vi "Configuração.vi"() -> ()   [LabVIEW 2018]
uses:
  Global_Telescopio.vi
panel:
  in  "URL do finals2000A.all:":string
  in  "Case Constant\n(See Context Help) 4":bool
  in  "Case Constant\n(See Context Help)":bool
  out "error out":errorcluster
  in  "Geral":T1(tab)=enum."Pos. Cúpula"
  in  "wheather timeout":bool
  in  "Tempo sem dados":dbl=120.0 caption="segundos" min=0.0
  in  "PressãoMax":dbl=1200.0 caption="mbar"
  in  "UmidadeMax":dbl=100.0 caption="%"
  in  "TemperaturaMax":dbl=30.0 caption="ºC"
  in  "PressãoMin":dbl=500.0 caption="mbar"
  in  "UmidadeMin":dbl caption="%"
  in  "TemperaturaMin":dbl caption="ºC"
  in  "Salvar valores":bool
  in  "Pressão atmosférica":dbl=880.0 caption="mbar"
  in  "Umidade":dbl=88.0 caption="%"
  in  "Temperatura":dbl=15.0 caption="ºC"
  in  "Default Met":bool
  in  "Memorizar Default Met":bool
  in  "Caminho Estação Meteorológica":string="V 1.0.0 arquivo obsoleto. Usado apenas PUB ZeroMQ."
  in  "Desloc_Min_Cúpula":i32=2 min=2
  in  "OffsetCupula":dbl=135.0 format="%#_11g"
  in  "Salvar dados cupula":bool
  in  "OffsetZ":dbl=-0.28 format="%#_11g"
  in  "OffsetY":dbl format="%#_11g"
  in  "OffsetX":dbl format="%#_11g"
  in  "DistEixos":dbl=-0.62 format="%#_11g"
  in  "RaioCup":dbl=3.2 format="%#_11g"
  in  "LATrad":dbl=5.889885056 format="%#_11g"
  in  "Conf. Serial":bool
  in  "Aquisição":i32(ring) items=[" COM1", " COM2", " COM3", " COM4", " COM5", " COM6", " COM7", " COM8", " COM9", " COM10", " COM11", " COM12", " COM13", " COM14", " COM15", " COM16", " COM17", " COM18", " COM19", " COM20"]
  in  "Guider":i32(ring) items=[" COM1", " COM2", " COM3", " COM4", " COM5", " COM6", " COM7", " COM8", " COM9", " COM10", " COM11", " COM12", " COM13", " COM14", " COM15", " COM16", " COM17", " COM18", " COM19", " COM20"]
  in  "Teclado":i32(ring) items=[" COM1", " COM2", " COM3", " COM4", " COM5", " COM6", " COM7", " COM8", " COM9", " COM10", " COM11", " COM12", " COM13", " COM14", " COM15", " COM16", " COM17", " COM18", " COM19", " COM20"]
  out "Calagem DEC":string
  out "Calagem AH":string
  in  "LoadCalagem":bool
  in  "Instrumento":u16(ring) items=["Coude A+", "Coude B+", "ECass+", "Eucalyptus+", "Cam 1+", "Cam 2*", "Cam4 + IV*", "Polarimetro*", "Fortrap*", "Cam1 RF*", "Coude C+", "MUSICOS*", "+Já testado", "* nao config", "cam 1 s/rf", "cam1srf/luca+focali", "Coude A/luca", "ECass/luca", "Cam1+rf+luca", "MUSICOS+Luca", "Camiv+Luca", "Cam2+Luca", "Cam1+rf+luca+Ixon", "Cam1+rf+luca+Ikon", "CoudeTeste"]
  in  "Conf. Instrumentos":bool
  in  "Tabela Instrumentos":string[][](table)=[["Coude", "281.52", " 11.53", "S", "S", "0.462", "23.1", "23.1"], ["Cassegrain", "281.52", " 11.53", "S", "S", "0.462", "23.1", "23.1"], ["Eucalyptus", "281.52", " 11.53", "S", "S", "0.462", "23.1", "23.1"], ["Cam 1", "281.52", " 11.53", "S", "S", "0.462", "23.1", "23.1"], ["Cam 2", "281.52", " 11.53", "S", "S", "0.462", "23.1", "23.1"], ["Cam IV", "281.52", " 11.53", "S", "S", "0.462", "23.1", "23.1"], ["Polarimetro", "281.52", " 11.53", "S", "S", "0.462", "23.1", "23.1"], ["Fortrap", "281.52", " 11.53", "S", "S", "0.462", "23.1", "23.1"]]
  in  "CorrecaoMin":dbl=0.1
  in  "tel_sts1":bool[](array[boolean])=[TRUE, TRUE, TRUE, TRUE, FALSE, FALSE, TRUE]
  in  "Senha LEAF":string
  in  "Enable ventilador":bool=TRUE
  in  "habilita supervisao":bool
  in  "Tempo delay":i32=1
  in  "Limite Oeste":dbl=5.0 min=-12.0 max=12.0 step=0.1
  in  "Limite Leste":dbl=-4.5 min=-12.0 max=12.0 step=0.1
  out "DownloadWait":bool
  out "DownloadOK":bool caption="OK"
  in  "Download_Finals2000A.all":bool
  in  "Tempo Atualização All Sky":i32=1 min=1
  in  "Tempo Atualização Cam 3":i32=1 min=1
  in  "Tempo Atualização Cam 2":i32=1 min=1
  in  "Tempo Atualização Cam 1":i32=1 min=1
  in  "Tempo Atualização Cam 0":i32=1 min=1
  out "Ângulo Zenital":dbl format="%#.1f"
  out "Azimute":dbl format="%#.1f"
  in  "Tabela Proteção":string[][](table)=[["0", "360", "70", "60", "65"]]
  in  "Raio Máximo":dbl=5.0 min=0.0 max=90.0 step=0.1
  in  "Z_Max":dbl
  in  "Z_Libera":dbl
  in  "Z_Segurança":dbl
  in  "Hour Angle":string="00 00 0,00" caption="Dest AH"
  in  "Dest Dec":string="00 00 00,00"
  in  "SALVA CONFIG":bool
  out "DestDEC":dbl
  in  "DestCUP":i32
  out "DestAH":dbl
  in  "Caminho camera":string
  in  "Hora vent inicial":i32=1 min=0 max=86399 step=1 format="%<%H:%M:%S>t"
  in  "Hora vent final":i32=1 min=0 max=86399 step=1 format="%<%H:%M:%S>t"
  in  "ENGENHARIA":bool
  # "Configuração do Sistema"
  # "Caminho completo da Estação Meteorológica\nEx: http://200.131.64.185/clima/download.txt"
  # "Especifica o tempo para sinalizar que o TCSPD não está\nrecebendo os dados da estação meteorológica."
  # "Usar valores default se ocorrer a sinalização descrita acima."
  # "Valores Médios"
  # "Limite Mínimo"
  # "Limite Máximo"
  # "Quando \"Default Met\" for selecionado, sempre serão usados os valores médios (default) de temperatura, umidade e pressão atmosférica no cálculo da refração atmostérica e não os valores lidos da estação meteorológica, mesmo que estes sejam válidos e corretos."
  # "Se alguma leitura da estação meteorológica estiver fora dos limites acima, aquele valor será automaticamente substituído pelo seu valor médio."
  # "CONSTANTES DA CÚPULA"
  # "1,60m"
  # "IAG"
  # "5,889885056"
  # "5,889885056"
  # "7,525"
  # "3,20"
  # "-0,62"
  # "1,570"
  # "0,000"
  # "0,000"
  # "0,000"
  # "0,000"
  # "0,300"
  # "-0,28"
  # "136,0"
  # "-135,0"
  # "4"
  # "2"
  # "Valores default para o IAG (03/03/2011)"
  # "Ao precionar as Teclas de Captura\né necessário selecionar  a Região \nde interesse da imagem!"
  # "Selecione a Captrua\na ser posicionada"
  # "Seriais\nAuto Guider"
  # "Ângulo\nRotator"
  # "Ângulo\nNorte"
  # "Img.\nEsp."
  # "No\nCass."
  # "Escala\nPlaca"
  # "Calagem\nAH (\")"
  # "Calagem\nDEC (\")"
  # "Posição\nFoco"
  # "Escolha do Instrumento"
  # "Instrumento"
  # "Calagem"
  # "Carrega a calagem do telescópio com a calagem inicial do instrumento"
  # "CorrecaoMin: Valor em arcsec utilizado como limite para mover os\neixos AH e DEC nos processos de guiagem automática (auto-guider)\ne de offset do sistema de aquisição. Não será executado nenhum \nmovimento desses processos com deslocamento inferior a CorrecaoMin."
  # "Parâmetros PARK"
  # "Radianos"
  # "-->"
  # "Faixa do Azimute\n   De:              Ate:"
  # "Ângulo Zenital\n  Máx:       Segur.:       Libera:"
  # "-->"
  # "Raio da Calagem Local"
  # "Graus"
  # "Tempo de delay de comunicação"
  # "Arquivo finals2000A.all para precessão"
  # "Habilita Supervisão do Controlador"
  # "Horas"
  # "Horas"
  # "C:\\TCS\\ARQUIVOS\\finals2000A.all,  2,2Mb"
  # "Ventilador"
  # "Endereço da câmera"
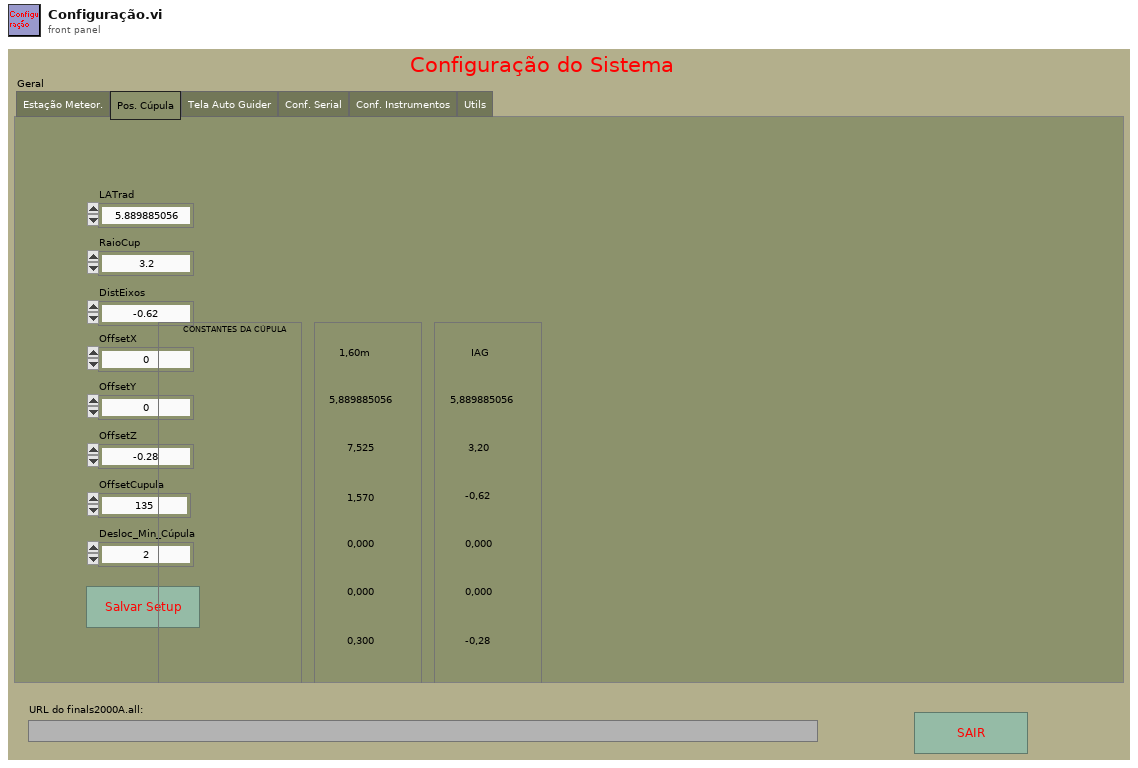
[diagram p1: front panel]
types:
  T1 = enum32{"Estação Meteor.", "Pos. Cúpula", "Tela Auto Guider", "Conf. Serial", "Conf. Instrumentos", "Utils"}
  T2 = cluster{"temperatura":dbl, "umidade":dbl, "pressao":dbl, "temperaturaMin":dbl, "umidadeMin":dbl, "pressaoMin":dbl, "temperaturaMax":dbl, "umidadeMax":dbl, "pressaoMax":dbl, "tempoSemDados":dbl}
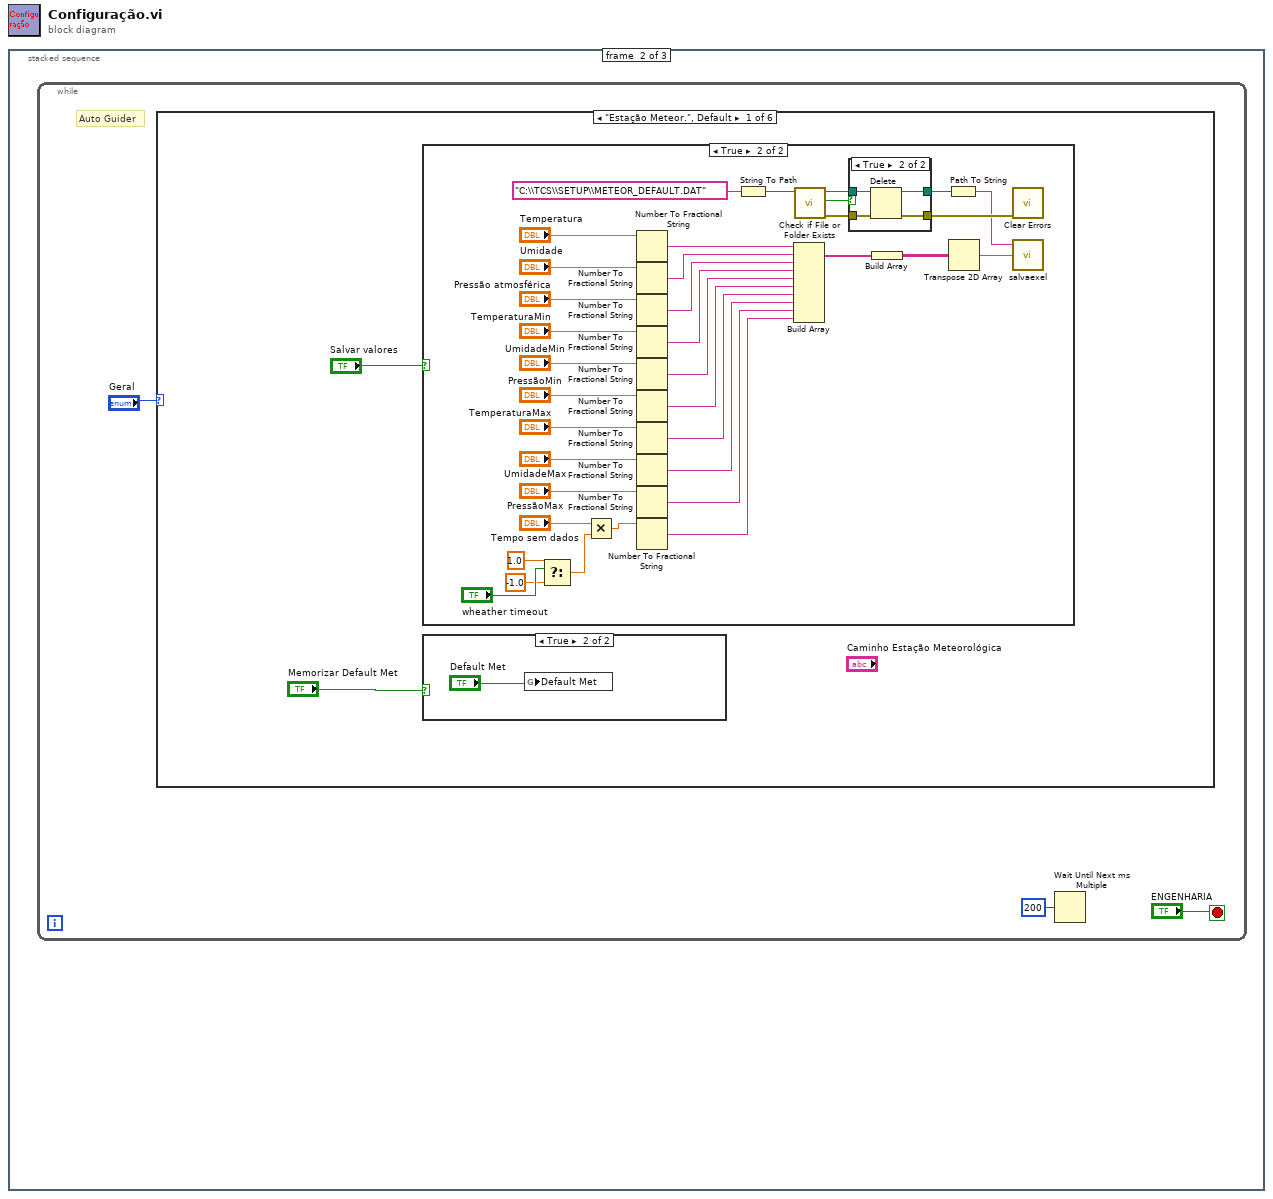
[diagram p0: block diagram]
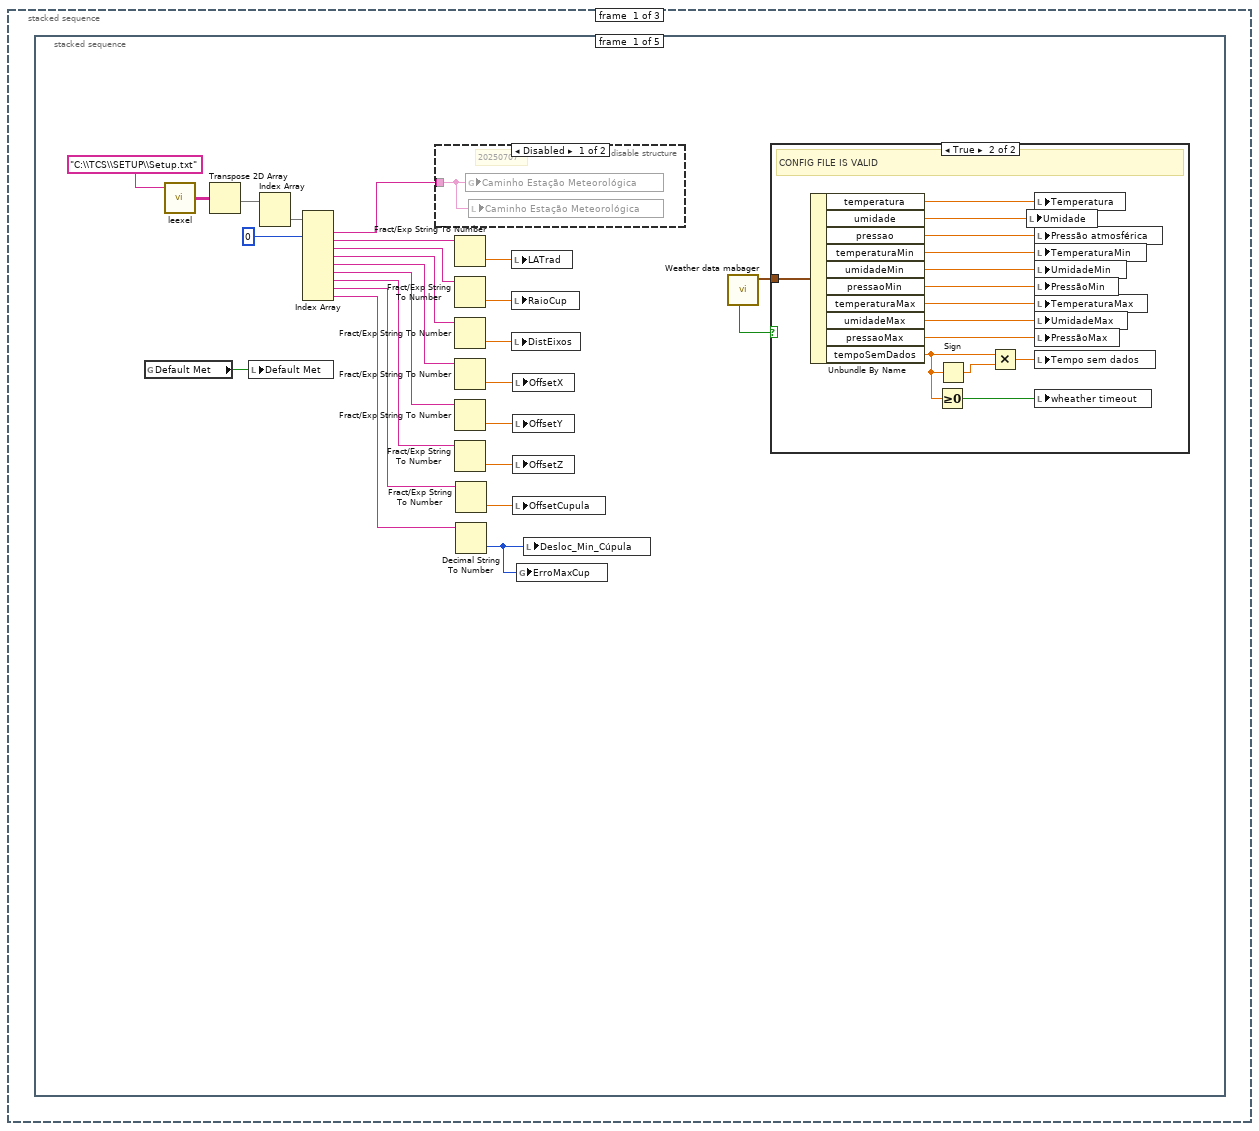
[diagram p2: hidden frame]
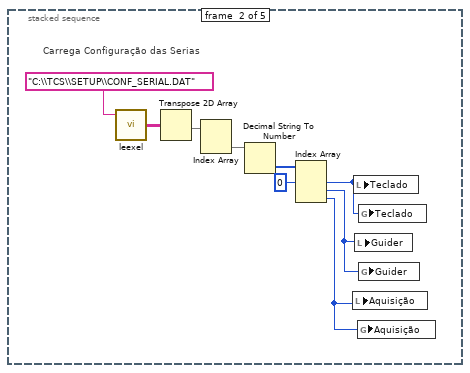
[diagram p5: hidden frame]
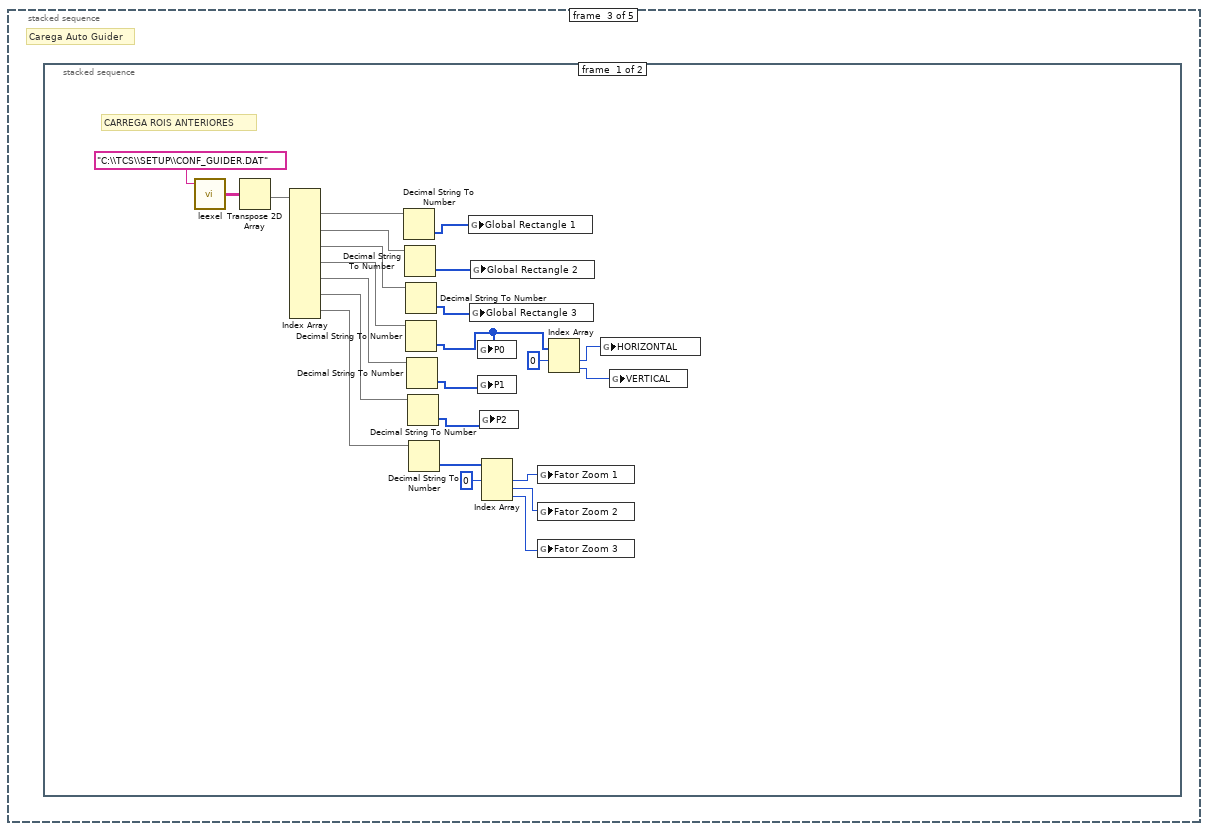
[diagram p6: hidden frame]
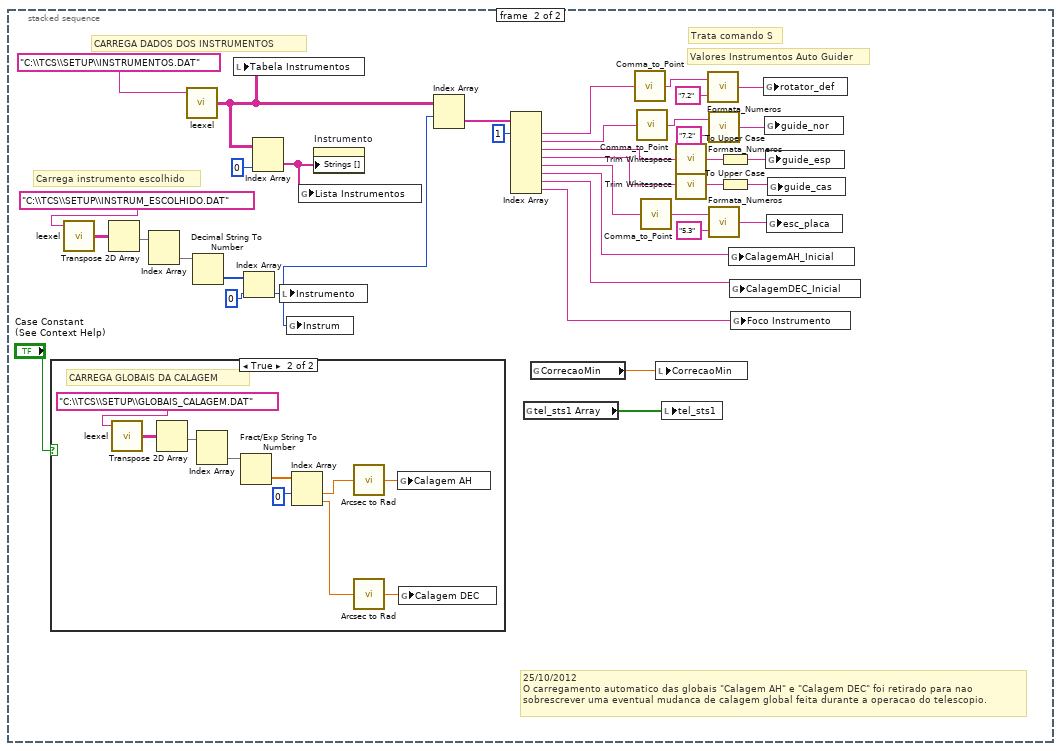
[diagram p7: hidden frame]
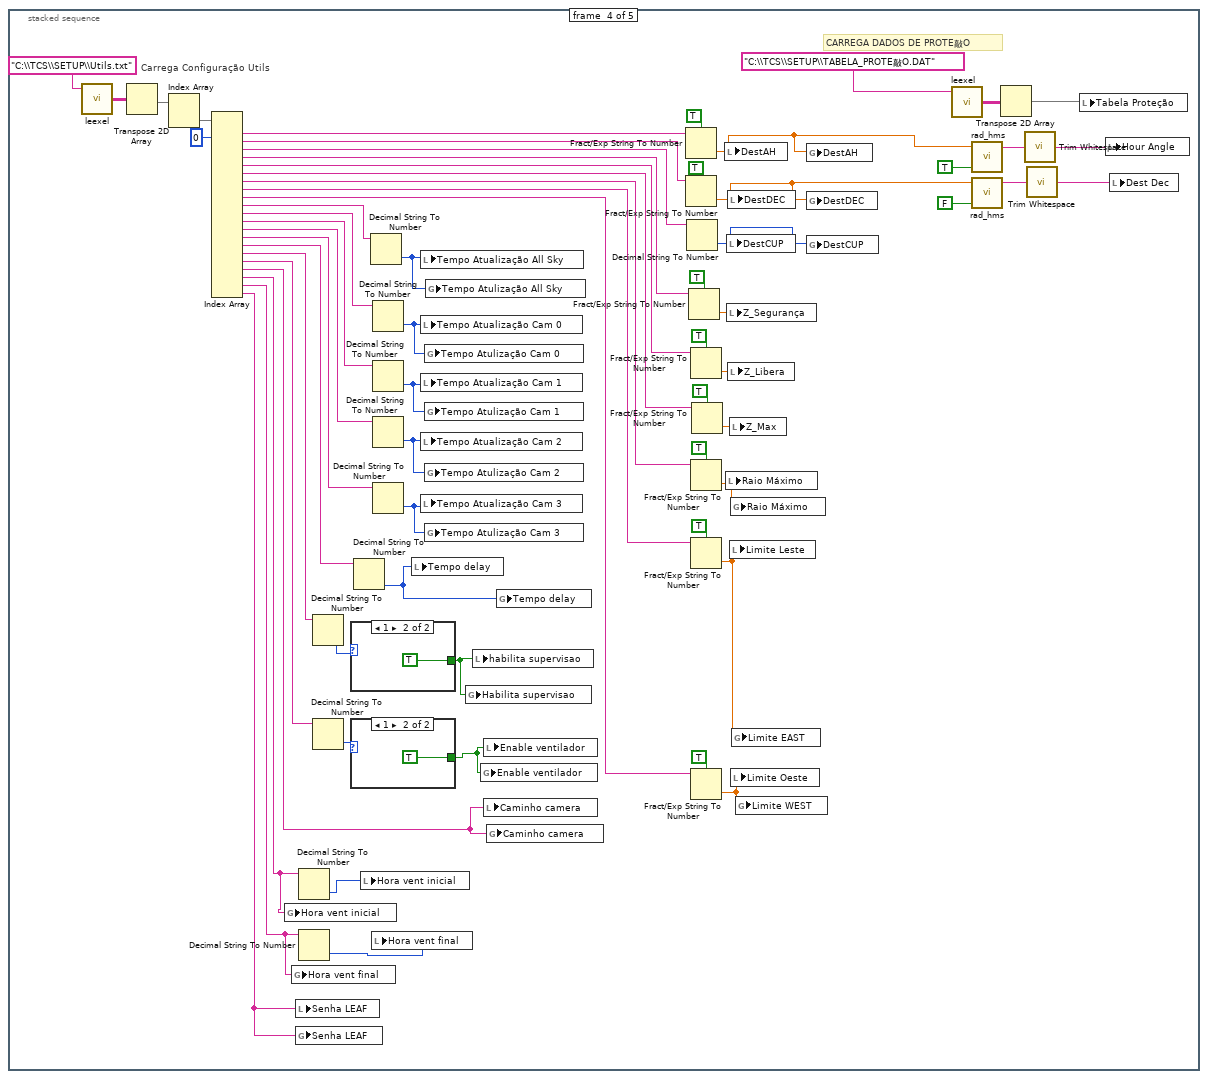
[diagram p9: hidden frame]
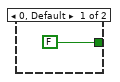
[diagram p10: hidden frame]
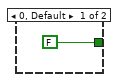
[diagram p11: hidden frame]
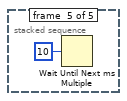
[diagram p12: hidden frame]
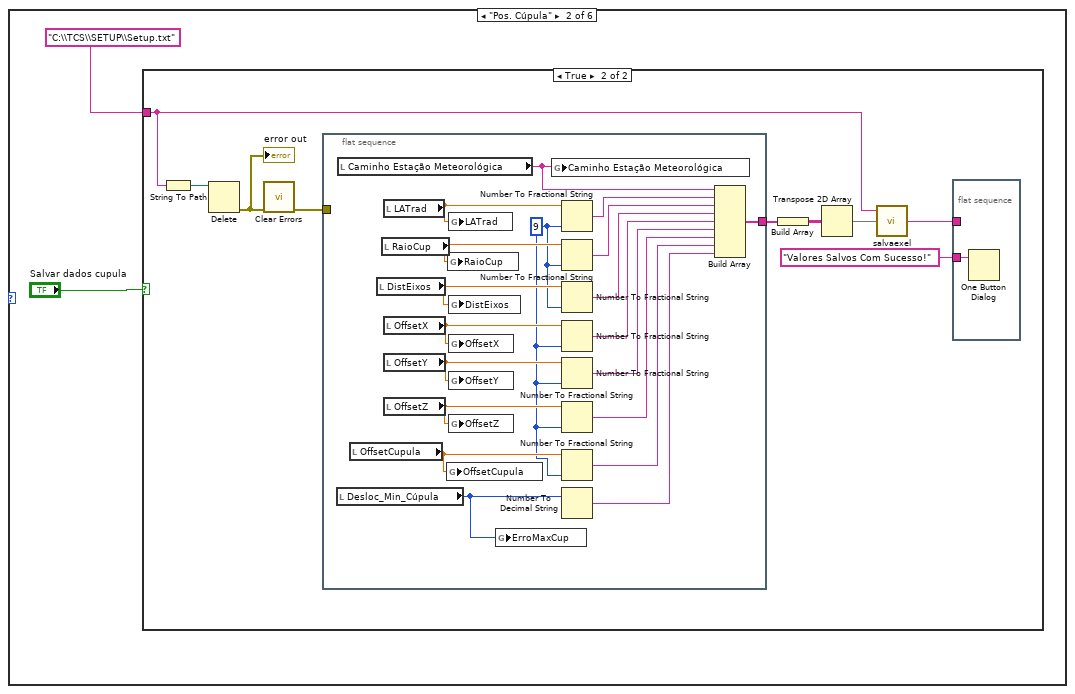
[diagram p16: hidden frame]
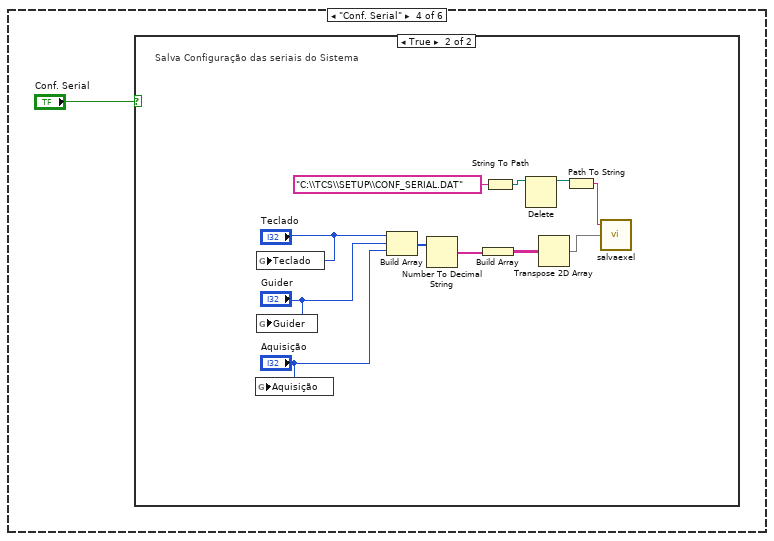
[diagram p19: hidden frame]
diagram:
  n1 = stacked-sequence {
    frame #0 {
      n2 = stacked-sequence {
        frame #0 {
          n3 = global read "Global_Telescopio.vi" "Default Met"() -> (w3:bool)
          n4 = call "leexel.vi"("path"="C:\\TCS\\SETUP\\Setup.txt") -> ("array 5"=w24:string[][])  [unwired: 4 in]
          n5 = Transpose 2D Array(2D array=w24) -> (transposed array=w23:string[][])
          n6 = local write "Default Met"(w3) -> ()
          n7 = Index Array(array=w23) -> (element=w22:string[])  [unwired: 2 in]
          n8 = Index Array(array=w22, index #1=0 ("index")) -> (element #1=w20:string, element #2=w18:string, element #3=w12:string, element #4=w11:string, element #5=w10:string, element #6=w9:string, element #7=w8:string, element #8=w6:string, element #9=w5:string)  [unwired: 8 in]
          n9 = disable-structure shown="Disabled" {
            disable-tunnel: w20 -> [w40 _]
            frame Disabled {
              # "20250707"
              n10 = global write "Global_Telescopio.vi" "Caminho Estação Meteorológica"(w40) -> ()
              n11 = local write "Caminho Estação Meteorológica"(w40) -> ()
            }
            frame Enabled {
            }
          }
          n12 = Fract/Exp String To Number(string=w18) -> (number=w19:dbl)  [unwired: 3 in, 1 out]
          n13 = Fract/Exp String To Number(string=w12) -> (number=w17:dbl)  [unwired: 3 in, 1 out]
          n14 = Fract/Exp String To Number(string=w11) -> (number=w16:dbl)  [unwired: 3 in, 1 out]
          n15 = Fract/Exp String To Number(string=w10) -> (number=w15:dbl)  [unwired: 3 in, 1 out]
          n16 = Fract/Exp String To Number(string=w9) -> (number=w14:dbl)  [unwired: 3 in, 1 out]
          n17 = Fract/Exp String To Number(string=w8) -> (number=w13:dbl)  [unwired: 3 in, 1 out]
          n18 = Fract/Exp String To Number(string=w6) -> (number=w7:dbl)  [unwired: 3 in, 1 out]
          n19 = Decimal String To Number(string=w5) -> (number=w4:i32)  [unwired: 2 in, 1 out]
          n20 = local write "LATrad"(w19) -> ()
          n21 = local write "RaioCup"(w17) -> ()
          n22 = local write "DistEixos"(w16) -> ()
          n23 = local write "OffsetX"(w15) -> ()
          n24 = local write "OffsetY"(w14) -> ()
          n25 = local write "OffsetZ"(w13) -> ()
          n26 = local write "OffsetCupula"(w7) -> ()
          n27 = global write "Global_Telescopio.vi" "ErroMaxCup"(w4) -> ()
          n28 = local write "Desloc_Min_Cúpula"(w4) -> ()
          n29 = call "Weather data mabager.vi"() -> ("weatherDefault"=w2:T2, "valid file"=w1:bool)  [unwired: 4 in, 6 out]
          n30 = case shown="True" w1 {
            tunnel: w2 -> [_ w39]
            frame False {
              # "INVALID CONFIG FILE - DOES NOT CHANGE DEFAULT CONTROL VALUES"
            }
            frame True {
              # "CONFIG FILE IS VALID"
              n31 = Unbundle By Name(w39) -> ("temperatura"=w38:dbl, "umidade"=w37:dbl, "pressao"=w36:dbl, "temperaturaMin"=w35:dbl, "umidadeMin"=w34:dbl, "pressaoMin"=w33:dbl, "temperaturaMax"=w32:dbl, "umidadeMax"=w31:dbl, "pressaoMax"=w30:dbl, "tempoSemDados"=w28:dbl)
              n32 = Greater Or Equal To 0?(x=w28) -> (x >= 0?=w29:bool)
              n33 = Sign(1:w28) -> (0:w27:dbl)
              n34 = Multiply(x=w28, y=w27) -> (x*y=w26:dbl)
              n35 = local write "Umidade"(w37) -> ()
              n36 = local write "Temperatura"(w38) -> ()
              n37 = local write "Pressão atmosférica"(w36) -> ()
              n38 = local write "TemperaturaMin"(w35) -> ()
              n39 = local write "UmidadeMin"(w34) -> ()
              n40 = local write "PressãoMin"(w33) -> ()
              n41 = local write "TemperaturaMax"(w32) -> ()
              n42 = local write "UmidadeMax"(w31) -> ()
              n43 = local write "PressãoMax"(w30) -> ()
              n44 = local write "Tempo sem dados"(w26) -> ()
              n45 = local write "wheather timeout"(w29) -> ()
            }
          }
        }
        frame #1 {
          # "Carrega Configuração das Serias"
          n46 = call "leexel.vi"("path"="C:\\TCS\\SETUP\\CONF_SERIAL.DAT") -> ("array 5"=w48:string[][])  [unwired: 4 in]
          n47 = Transpose 2D Array(2D array=w48) -> (transposed array=w47:string[][])
          n48 = Index Array(array=w47) -> (element=w49:string[])  [unwired: 2 in]
          n49 = Decimal String To Number(string=w49) -> (number=w45:i32[])  [unwired: 2 in, 1 out]
          n50 = Index Array(array=w45, index #1=0 ("index")) -> (element #1=w43:i32, element #2=w42:i32, element #3=w41:i32)  [unwired: 2 in]
          n51 = local write "Aquisição"(w41) -> ()
          n52 = local write "Teclado"(w43) -> ()
          n53 = local write "Guider"(w42) -> ()
          n54 = global write "Global_Telescopio.vi" "Aquisição"(w41) -> ()
          n55 = global write "Global_Telescopio.vi" "Teclado"(w43) -> ()
          n56 = global write "Global_Telescopio.vi" "Guider"(w42) -> ()
        }
        frame #2 {
          # "Carega Auto Guider"
          n57 = stacked-sequence {
            frame #0 {
              # "CARREGA ROIS ANTERIORES"
              n58 = call "leexel.vi"("path"="C:\\TCS\\SETUP\\CONF_GUIDER.DAT") -> ("array 5"=w72:string[][])  [unwired: 4 in]
              n59 = Transpose 2D Array(2D array=w72) -> (transposed array=w71:string[][])
              n60 = Index Array(array=w71) -> (element #1=w70:string[], element #2=w69:string[], element #3=w68:string[], element #4=w67:string[], element #5=w66:string[], element #6=w65:string[], element #7=w53:string[])  [unwired: 14 in]
              n61 = Decimal String To Number(string=w70) -> (number=w56:i32[])  [unwired: 2 in, 1 out]
              n62 = Decimal String To Number(string=w69) -> (number=w57:i32[])  [unwired: 2 in, 1 out]
              n63 = Decimal String To Number(string=w68) -> (number=w58:i32[])  [unwired: 2 in, 1 out]
              n64 = Decimal String To Number(string=w67) -> (number=w61:i32[])  [unwired: 2 in, 1 out]
              n65 = Decimal String To Number(string=w66) -> (number=w60:i32[])  [unwired: 2 in, 1 out]
              n66 = Decimal String To Number(string=w65) -> (number=w59:i32[])  [unwired: 2 in, 1 out]
              n67 = Decimal String To Number(string=w53) -> (number=w52:i32[])  [unwired: 2 in, 1 out]
              n68 = global write "Global_Telescopio.vi" "Global Rectangle 1"(w56) -> ()
              n69 = global write "Global_Telescopio.vi" "Global Rectangle 3"(w58) -> ()
              n70 = global write "Global_Telescopio.vi" "Global Rectangle 2"(w57) -> ()
              n71 = global write "Global_Telescopio.vi" "P0"(w61) -> ()
              n72 = global write "Global_Telescopio.vi" "P1"(w60) -> ()
              n73 = global write "Global_Telescopio.vi" "P2"(w59) -> ()
              n74 = Index Array(array=w52, index #1=0 ("index")) -> (element #1=w54:i32, element #2=w51:i32, element #3=w50:i32)  [unwired: 2 in]
              n75 = global write "Global_Telescopio.vi" "Fator Zoom 1"(w54) -> ()
              n76 = global write "Global_Telescopio.vi" "Fator Zoom 2"(w51) -> ()
              n77 = global write "Global_Telescopio.vi" "Fator Zoom 3"(w50) -> ()
              n78 = Index Array(array=w61, index #1=0 ("index")) -> (element #1=w63:i32, element #2=w62:i32)  [unwired: 1 in]
              n79 = global write "Global_Telescopio.vi" "HORIZONTAL"(w63) -> ()
              n80 = global write "Global_Telescopio.vi" "VERTICAL"(w62) -> ()
            }
            frame #1 {
              # "25/10/2012\nO carregamento automatico das globais \"Calagem AH\" e \"Calagem DEC\" foi retirado para nao \nsobrescrever uma eventual mudanca de calagem global feita durante a operacao do telescopio."
              # "Trata comando S"
              # "Valores Instrumentos Auto Guider"
              # "Carrega instrumento escolhido"
              # "CARREGA DADOS DOS INSTRUMENTOS"
              n81 = case shown="True" "Case Constant\n(See Context Help)" {
                frame False {
                }
                frame True {
                  # "CARREGA GLOBAIS DA CALAGEM"
                  n82 = call "leexel.vi"("path"="C:\\TCS\\SETUP\\GLOBAIS_CALAGEM.DAT") -> ("array 5"=w117:string[][])  [unwired: 4 in]
                  n83 = Transpose 2D Array(2D array=w117) -> (transposed array=w118:string[][])
                  n84 = Index Array(array=w118) -> (element=w116:string[])  [unwired: 2 in]
                  n85 = Fract/Exp String To Number(string=w116) -> (number=w120:dbl[])  [unwired: 3 in, 1 out]
                  n86 = Index Array(array=w120, index #1=0 ("index")) -> (element #1=w114:dbl, element #2=w113:dbl)  [unwired: 1 in]
                  n87 = call "Arcsec to Rad.vi"("Arcsec"=w114) -> ("rad"=w112:dbl)
                  n88 = call "Arcsec to Rad.vi"("Arcsec"=w113) -> ("rad"=w111:dbl)
                  n89 = global write "Global_Telescopio.vi" "Calagem AH"(w112) -> ()
                  n90 = global write "Global_Telescopio.vi" "Calagem DEC"(w111) -> ()
                }
              }
              n91 = call "leexel.vi"("path"="C:\\TCS\\SETUP\\INSTRUM_ESCOLHIDO.DAT") -> ("array 5"=w106:string[][])  [unwired: 4 in]
              n92 = Transpose 2D Array(2D array=w106) -> (transposed array=w105:string[][])
              n93 = Index Array(array=w105) -> (element=w107:string[])  [unwired: 2 in]
              n94 = call "leexel.vi"("path"="C:\\TCS\\SETUP\\INSTRUMENTOS.DAT") -> ("array 5"=w102:string[][])  [unwired: 4 in]
              n95 = Decimal String To Number(string=w107) -> (number=w103:i32[])  [unwired: 2 in, 1 out]
              n96 = local write "Tabela Instrumentos"(w102) -> ()
              n97 = Index Array(array=w103, index=0) -> (element=w94:i32)
              n98 = Index Array(array=w102, index (col)=0 ("disabled index (col)")) -> (element=w95:string[])  [unwired: 1 in]
              n99 = local write "Instrumento"(w94) -> ()
              n100 = global write "Global_Telescopio.vi" "Instrum"(w94) -> ()
              n101 = global write "Global_Telescopio.vi" "Lista Instrumentos"(w95) -> ()
              n102 = property on="Instrumento" class="Ring (strict)"("Strings []"=w95) -> ()  [unwired: 2 in, 2 out]
              n103 = Index Array(array=w102, index (row)=w94) -> (element=w100:string[])  [unwired: 1 in]
              n104 = Index Array(array=w100, index #1=1 ("index")) -> (element #1=w90:string, element #2=w86:string, element #3=w83:string, element #4=w80:string, element #5=w76:string, element #6=w97:string, element #7=w96:string, element #8=w75:string)  [unwired: 7 in]
              n105 = global read "Global_Telescopio.vi" "tel_sts1 Array"() -> (w98:bool[])
              n106 = global read "Global_Telescopio.vi" "CorrecaoMin"() -> (w99:dbl)
              n107 = call "Comma_to_Point.vi"("Lat_A"=w90) -> ("Saída"=w91:string)
              n108 = call "Comma_to_Point.vi"("Lat_A"=w86) -> ("Saída"=w87:string)
              n109 = call "Comma_to_Point.vi"("Lat_A"=w76) -> ("Saída"=w77:string)
              n110 = local write "CorrecaoMin"(w99) -> ()
              n111 = local write "tel_sts1"(w98) -> ()
              n112 = call <vilib>:"Trim Whitespace.vi"("string"=w83) -> ("trimmed string"=w85:string)  [unwired: 1 in]
              n113 = call <vilib>:"Trim Whitespace.vi"("string"=w80) -> ("trimmed string"=w82:string)  [unwired: 1 in]
              n114 = call "Formata_Numeros.vi"("Formato ex-> 7.2"="7.2", "Valor num"=w91) -> ("resulting string"=w92:string)
              n115 = call "Formata_Numeros.vi"("Formato ex-> 7.2"="7.2", "Valor num"=w87) -> ("resulting string"=w88:string)
              n116 = call "Formata_Numeros.vi"("Formato ex-> 7.2"="5.3", "Valor num"=w77) -> ("resulting string"=w78:string)
              n117 = To Upper Case(1:w85) -> (0:w84:string)
              n118 = To Upper Case(1:w82) -> (0:w81:string)
              n119 = global write "Global_Telescopio.vi" "CalagemAH_Inicial"(w97) -> ()
              n120 = global write "Global_Telescopio.vi" "CalagemDEC_Inicial"(w96) -> ()
              n121 = global write "Global_Telescopio.vi" "Foco Instrumento"(w75) -> ()
              n122 = global write "Global_Telescopio.vi" "rotator_def"(w92) -> ()
              n123 = global write "Global_Telescopio.vi" "guide_nor"(w88) -> ()
              n124 = global write "Global_Telescopio.vi" "guide_esp"(w84) -> ()
              n125 = global write "Global_Telescopio.vi" "esc_placa"(w78) -> ()
              n126 = global write "Global_Telescopio.vi" "guide_cas"(w81) -> ()
            }
          }
        }
        frame #3 {
          # "CARREGA DADOS DE PROTE敲O"
          # "Carrega Configuração Utils"
          n127 = call "leexel.vi"("path"="C:\\TCS\\SETUP\\Utils.txt") -> ("array 5"=w183:string[][])  [unwired: 4 in]
          n128 = Transpose 2D Array(2D array=w183) -> (transposed array=w182:string[][])
          n129 = Index Array(array=w182) -> (element=w181:string[])  [unwired: 2 in]
          n130 = Index Array(array=w181, index #1=0 ("index")) -> (element #1=w179:string, element #2=w178:string, element #3=w177:string, element #4=w162:string, element #5=w161:string, element #6=w160:string, element #7=w154:string, element #8=w136:string, element #9=w135:string, element #10=w141:string, element #11=w142:string, element #12=w143:string, element #13=w144:string, element #14=w145:string, element #15=w134:string, element #16=w133:string, element #17=w126:string, element #18=w127:string, element #19=w122:string, element #20=w123:string, element #21=w121:string)  [unwired: 20 in]
          n131 = global write "Global_Telescopio.vi" "Hora vent inicial"(w122) -> ()
          n132 = global write "Global_Telescopio.vi" "Hora vent final"(w123) -> ()
          n133 = local write "Senha LEAF"(w121) -> ()
          n134 = global write "Global_Telescopio.vi" "Senha LEAF"(w121) -> ()
          n135 = Decimal String To Number(string=w122) -> (number=w125:i32)  [unwired: 2 in, 1 out]
          n136 = Decimal String To Number(string=w123) -> (number=w124:i32)  [unwired: 2 in, 1 out]
          n137 = Decimal String To Number(string=w133) -> (number=w132:i32)  [unwired: 2 in, 1 out]
          n138 = Decimal String To Number(string=w126) -> (number=w129:i32)  [unwired: 2 in, 1 out]
          n139 = case shown="1" w132 {
            tunnel: [FALSE TRUE] -> w131
            frame 0, Default {
            }
            frame 1 {
            }
          }
          n140 = case shown="1" w129 {
            tunnel: [FALSE TRUE] -> w128
            frame 0, Default {
            }
            frame 1 {
            }
          }
          n141 = Decimal String To Number(string=w134) -> (number=w130:i32)  [unwired: 2 in, 1 out]
          n142 = local write "Hora vent inicial"(w125) -> ()
          n143 = Decimal String To Number(string=w141) -> (number=w150:i32)  [unwired: 2 in, 1 out]
          n144 = local write "Hora vent final"(w124) -> ()
          n145 = Decimal String To Number(string=w142) -> (number=w149:i32)  [unwired: 2 in, 1 out]
          n146 = Decimal String To Number(string=w143) -> (number=w148:i32)  [unwired: 2 in, 1 out]
          n147 = Decimal String To Number(string=w144) -> (number=w147:i32)  [unwired: 2 in, 1 out]
          n148 = Decimal String To Number(string=w145) -> (number=w146:i32)  [unwired: 2 in, 1 out]
          n149 = local write "Tempo delay"(w130) -> ()
          n150 = local write "Tempo Atualização All Sky"(w150) -> ()
          n151 = local write "Tempo Atualização Cam 0"(w149) -> ()
          n152 = local write "Tempo Atualização Cam 1"(w148) -> ()
          n153 = local write "Tempo Atualização Cam 2"(w147) -> ()
          n154 = local write "Tempo Atualização Cam 3"(w146) -> ()
          n155 = global write "Global_Telescopio.vi" "Tempo Atulização Cam 0"(w149) -> ()
          n156 = global write "Global_Telescopio.vi" "Tempo Atulização Cam 1"(w148) -> ()
          n157 = global write "Global_Telescopio.vi" "Tempo Atulização Cam 2"(w147) -> ()
          n158 = global write "Global_Telescopio.vi" "Tempo Atulização Cam 3"(w146) -> ()
          n159 = global write "Global_Telescopio.vi" "Tempo Atulização All Sky"(w150) -> ()
          n160 = global write "Global_Telescopio.vi" "Habilita supervisao"(w131) -> ()
          n161 = local write "habilita supervisao"(w131) -> ()
          n162 = global write "Global_Telescopio.vi" "Enable ventilador"(w128) -> ()
          n163 = local write "Enable ventilador"(w128) -> ()
          n164 = local write "Caminho camera"(w127) -> ()
          n165 = global write "Global_Telescopio.vi" "Caminho camera"(w127) -> ()
          n166 = global write "Global_Telescopio.vi" "Tempo delay"(w130) -> ()
          n167 = Fract/Exp String To Number(use system decimal point (T)=TRUE, string=w179) -> (number=w173:dbl)  [unwired: 2 in, 1 out]
          n168 = Fract/Exp String To Number(use system decimal point (T)=TRUE, string=w178) -> (number=w172:dbl)  [unwired: 2 in, 1 out]
          n169 = Decimal String To Number(string=w177) -> (number=w176:i32)  [unwired: 2 in, 1 out]
          n170 = Fract/Exp String To Number(use system decimal point (T)=TRUE, string=w162) -> (number=w159:dbl)  [unwired: 2 in, 1 out]
          n171 = Fract/Exp String To Number(use system decimal point (T)=TRUE, string=w161) -> (number=w158:dbl)  [unwired: 2 in, 1 out]
          n172 = Fract/Exp String To Number(use system decimal point (T)=TRUE, string=w154) -> (number=w155:dbl)  [unwired: 2 in, 1 out]
          n173 = Fract/Exp String To Number(use system decimal point (T)=TRUE, string=w136) -> (number=w137:dbl)  [unwired: 2 in, 1 out]
          n174 = Fract/Exp String To Number(use system decimal point (T)=TRUE, string=w135) -> (number=w138:dbl)  [unwired: 2 in, 1 out]
          n175 = Fract/Exp String To Number(use system decimal point (T)=TRUE, string=w160) -> (number=w157:dbl)  [unwired: 2 in, 1 out]
          n176 = local write "DestAH"(w173) -> ()
          n177 = local write "Raio Máximo"(w155) -> ()
          n178 = local write "DestCUP"(w176) -> ()
          n179 = local write "Z_Segurança"(w159) -> ()
          n180 = local write "DestDEC"(w172) -> ()
          n181 = local write "Z_Libera"(w158) -> ()
          n182 = local write "Z_Max"(w157) -> ()
          n183 = local write "Limite Leste"(w137) -> ()
          n184 = global write "Global_Telescopio.vi" "Raio Máximo"(w155) -> ()
          n185 = local write "Limite Oeste"(w138) -> ()
          n186 = global write "Global_Telescopio.vi" "Limite EAST"(w137) -> ()
          n187 = global write "Global_Telescopio.vi" "Limite WEST"(w138) -> ()
          n188 = global write "Global_Telescopio.vi" "DestAH"(w173) -> ()
          n189 = global write "Global_Telescopio.vi" "DestDEC"(w172) -> ()
          n190 = global write "Global_Telescopio.vi" "DestCUP"(w176) -> ()
          n191 = call "leexel.vi"("path"="C:\\TCS\\SETUP\\TABELA_PROTE敲O.DAT") -> ("array 5"=w152:string[][])  [unwired: 4 in]
          n192 = call "rad_hms.vi"("TRUE=HORA\nFALSE=GRAU"=TRUE, "Radiano"=w173) -> ("Hora/Graus Texto Decimal"=w167:string)  [unwired: 3 in]
          n193 = call "rad_hms.vi"("TRUE=HORA\nFALSE=GRAU"=FALSE, "Radiano"=w172) -> ("Hora/Graus Texto Decimal"=w166:string)  [unwired: 3 in]
          n194 = Transpose 2D Array(2D array=w152) -> (transposed array=w151:string[][])
          n195 = call <vilib>:"Trim Whitespace.vi"("string"=w167) -> ("trimmed string"=w168:string)  [unwired: 1 in]
          n196 = call <vilib>:"Trim Whitespace.vi"("string"=w166) -> ("trimmed string"=w169:string)  [unwired: 1 in]
          n197 = local write "Tabela Proteção"(w151) -> ()
          n198 = local write "Hour Angle"(w168) -> ()
          n199 = local write "Dest Dec"(w169) -> ()
        }
        frame #4 {
          n200 = Wait Until Next ms Multiple(millisecond multiple=u32 10) -> ()  [unwired: 1 out]
        }
      }
    }
    frame #1 {
      n201 = while {
        stop <- "ENGENHARIA" stop-if-true
        # "Auto Guider"
        n202 = case shown="\"Estação Meteor.\", Default" "Geral" {
          frame "Estação Meteor.", Default {
            n203 = case shown="True" "Salvar valores" {
              frame False {
              }
              frame True {
                n204 = Select(t=1.0, s="wheather timeout", f=-1.0 ("t")) -> (s? t:f=w198:dbl)
                n205 = Multiply(x="Tempo sem dados", y=w198) -> (x*y=w200:dbl)
                n206 = Number To Fractional String(number="Temperatura") -> (F-format string=w229:string)  [unwired: 3 in]
                n207 = Number To Fractional String(number="Umidade") -> (F-format string=w228:string)  [unwired: 3 in]
                n208 = Number To Fractional String(number="Pressão atmosférica") -> (F-format string=w227:string)  [unwired: 3 in]
                n209 = Number To Fractional String(number="TemperaturaMin") -> (F-format string=w207:string)  [unwired: 3 in]
                n210 = Number To Fractional String(number="UmidadeMin") -> (F-format string=w206:string)  [unwired: 3 in]
                n211 = Number To Fractional String(number="PressãoMin") -> (F-format string=w205:string)  [unwired: 3 in]
                n212 = Number To Fractional String(number="TemperaturaMax") -> (F-format string=w204:string)  [unwired: 3 in]
                n213 = Number To Fractional String(number="UmidadeMax") -> (F-format string=w203:string)  [unwired: 3 in]
                n214 = Number To Fractional String(number="PressãoMax") -> (F-format string=w202:string)  [unwired: 3 in]
                n215 = Number To Fractional String(number=w200) -> (F-format string=w201:string)  [unwired: 3 in]
                n216 = String To Path(string="C:\\TCS\\SETUP\\METEOR_DEFAULT.DAT") -> (path=w220:path)
                n217 = Build Array(w229, w228, w227, w207, w206, w205, w204, w203, w202, w201) -> (w223:string[])
                n218 = call <vilib>:"Check if File or Folder Exists.vi"("path"=w220) -> ("error out"=w218:errorcluster, "file or folder exists?"=w217:bool, "dup path"=w219:path)  [unwired: 8 in]
                n219 = case shown="True" w217 {
                  tunnel: [w231 w236] -> w221
                  tunnel: w219 -> [w232 w235]
                  tunnel: w218 -> [w231 w234]
                  tunnel: [w232 w233] -> w216
                  frame False {
                  }
                  frame True {
                    n220 = Delete(path (use dialog)=w235, error in=w234) -> (deleted path=w233:path, error out=w236:errorcluster)  [unwired: 3 in, 1 out]
                  }
                }
                n221 = Build Array(w223) -> (w222:string[][])
                n222 = Path To String(path=w216) -> (string=w214:string)
                n223 = Transpose 2D Array(2D array=w222) -> (transposed array=w230:string[][])
                n224 = call <vilib>:"Clear Errors.vi"("error in (no error)"=w221) -> ()  [unwired: 5 in, 2 out]
                n225 = call "salvaexel.vi"("appended array"=w230, "file name p/ exell"=w214) -> ()  [unwired: 1 in, 1 out]
              }
            }
            n226 = case shown="True" "Memorizar Default Met" {
              frame False {
              }
              frame True {
                n227 = global write "Global_Telescopio.vi" "Default Met"("Default Met") -> ()
              }
            }
          }
          frame "Pos. Cúpula" {
            n228 = case shown="True" "Salvar dados cupula" {
              tunnel: "C:\\TCS\\SETUP\\Setup.txt" -> [_ w242]
              frame False {
              }
              frame True {
                n229 = String To Path(string=w242) -> (path=w248:path)
                n230 = Delete(path (use dialog)=w248) -> (error out=w247:errorcluster)  [unwired: 4 in, 2 out]
                "error out" <- w247
                n231 = call <vilib>:"Clear Errors.vi"("error in (no error)"=w247) -> ("error out"=w246:errorcluster)  [unwired: 5 in, 1 out]
                n232 = flat-sequence {
                  tunnel: w246 -> [_]
                  tunnel: [w251] -> w243
                  frame #0 {
                    w252 = i16 9 ("precision (6)")
                    n233 = local read "Desloc_Min_Cúpula"() -> (w260:i32)
                    n234 = local read "Caminho Estação Meteorológica"() -> (w250:string)
                    n235 = local read "OffsetCupula"() -> (w253:dbl)
                    n236 = local read "DistEixos"() -> (w257:dbl)
                    n237 = local read "RaioCup"() -> (w258:dbl)
                    n238 = local read "LATrad"() -> (w259:dbl)
                    n239 = local read "OffsetX"() -> (w256:dbl)
                    n240 = local read "OffsetY"() -> (w255:dbl)
                    n241 = local read "OffsetZ"() -> (w254:dbl)
                    n242 = global write "Global_Telescopio.vi" "OffsetCupula"(w253) -> ()
                    n243 = global write "Global_Telescopio.vi" "RaioCup"(w258) -> ()
                    n244 = global write "Global_Telescopio.vi" "LATrad"(w259) -> ()
                    n245 = global write "Global_Telescopio.vi" "DistEixos"(w257) -> ()
                    n246 = global write "Global_Telescopio.vi" "OffsetX"(w256) -> ()
                    n247 = global write "Global_Telescopio.vi" "OffsetY"(w255) -> ()
                    n248 = global write "Global_Telescopio.vi" "OffsetZ"(w254) -> ()
                    n249 = global write "Global_Telescopio.vi" "ErroMaxCup"(w260) -> ()
                    n250 = global write "Global_Telescopio.vi" "Caminho Estação Meteorológica"(w250) -> ()
                    n251 = Number To Fractional String(number=w259, precision (6)=w252) -> (F-format string=w268:string)  [unwired: 2 in]
                    n252 = Number To Fractional String(number=w258, precision (6)=w252) -> (F-format string=w267:string)  [unwired: 2 in]
                    n253 = Number To Fractional String(number=w257, precision (6)=w252) -> (F-format string=w266:string)  [unwired: 2 in]
                    n254 = Number To Fractional String(number=w256, precision (6)=w252) -> (F-format string=w265:string)  [unwired: 2 in]
                    n255 = Number To Fractional String(number=w255, precision (6)=w252) -> (F-format string=w264:string)  [unwired: 2 in]
                    n256 = Number To Fractional String(number=w254, precision (6)=w252) -> (F-format string=w263:string)  [unwired: 2 in]
                    n257 = Number To Fractional String(number=w253, precision (6)=w252) -> (F-format string=w262:string)  [unwired: 2 in]
                    n258 = Number To Decimal String(number=w260) -> (decimal integer string=w261:string)  [unwired: 1 in]
                    n259 = Build Array(w250, w268, w267, w266, w265, w264, w263, w262, w261) -> (w251:string[])
                  }
                }
                n260 = Build Array(w243) -> (w245:string[][])
                n261 = Transpose 2D Array(2D array=w245) -> (transposed array=w244:string[][])
                n262 = call "salvaexel.vi"("appended array"=w244, "file name p/ exell"=w242) -> ("spreadsheet string"=w240:string)  [unwired: 1 in]
                n263 = flat-sequence {
                  tunnel: "Valores Salvos Com Sucesso!" ("message") -> [w249]
                  tunnel: w240 -> [_]
                  frame #0 {
                    n264 = One Button Dialog(message=w249) -> ()  [unwired: 1 in, 1 out]
                  }
                }
              }
            }
          }
          frame "Tela Auto Guider" {
          }
          frame "Conf. Serial" {
            n265 = case shown="True" "Conf. Serial" {
              frame False {
              }
              frame True {
                # "Salva Configuração das seriais do Sistema"
                n266 = global write "Global_Telescopio.vi" "Aquisição"("Aquisição") -> ()
                n267 = global write "Global_Telescopio.vi" "Teclado"("Teclado") -> ()
                n268 = global write "Global_Telescopio.vi" "Guider"("Guider") -> ()
                n269 = Build Array("Teclado", "Guider", "Aquisição") -> (w280:i32[])
                n270 = Number To Decimal String(number=w280) -> (decimal integer string=w270:string[])  [unwired: 1 in]
                n271 = Build Array(w270) -> (w275:string[][])
                n272 = String To Path(string="C:\\TCS\\SETUP\\CONF_SERIAL.DAT") -> (path=w273:path)
                n273 = Delete(path (use dialog)=w273) -> (deleted path=w272:path)  [unwired: 4 in, 2 out]
                n274 = Transpose 2D Array(2D array=w275) -> (transposed array=w274:string[][])
                n275 = Path To String(path=w272) -> (string=w271:string)
                n276 = call "salvaexel.vi"("appended array"=w274, "file name p/ exell"=w271) -> ()  [unwired: 1 in, 1 out]
              }
            }
          }
          frame "Conf. Instrumentos" {
            n277 = stacked-sequence {
              frame #0 {
                w283 = i16 1 ("precision (6)")
                n278 = global read "Global_Telescopio.vi" "Calagem AH"() -> (w284:dbl)
                n279 = global read "Global_Telescopio.vi" "Calagem DEC"() -> (w287:dbl)
                n280 = local read "Tabela Instrumentos"() -> (w291:string[][])
                n281 = call "Rad to Arcsec.vi"("Radiano"=w287) -> ("Arcsec"=w286:dbl)
                n282 = call "Rad to Arcsec.vi"("Radiano"=w284) -> ("Arcsec"=w285:dbl)
                n283 = Number To Fractional String(number=w286, precision (6)=w283) -> (F-format string=→"Calagem DEC":string)  [unwired: 2 in]
                n284 = Number To Fractional String(number=w285, precision (6)=w283) -> (F-format string=→"Calagem AH":string)  [unwired: 2 in]
                n285 = Index Array(array=w291, index (col)=0 ("disabled index (col)")) -> (element=w289:string[])  [unwired: 1 in]
                n286 = property on="Instrumento" class="Ring (strict)"("Strings []"=w289) -> ()  [unwired: 2 in, 2 out]
                n287 = case shown="True" "LoadCalagem" {
                  selector: "LoadCalagem" -> [_ w294]
                  frame False {
                  }
                  frame True {
                    # "Faz a Calagem do telescópio igual à calagem inicial do instrumento"
                    n288 = global read "Global_Telescopio.vi" "CalagemDEC_Inicial"() -> (w296:string)
                    n289 = global read "Global_Telescopio.vi" "CalagemAH_Inicial"() -> (w300:string)
                    n290 = global write "Global_Telescopio.vi" "Flag-Rotator"(w294) -> ()
                    n291 = Fract/Exp String To Number(string=w300) -> (number=w299:dbl)  [unwired: 3 in, 1 out]
                    n292 = Fract/Exp String To Number(string=w296) -> (number=w297:dbl)  [unwired: 3 in, 1 out]
                    n293 = call "Arcsec to Rad.vi"("Arcsec"=w299) -> ("rad"=w298:dbl)
                    n294 = call "Arcsec to Rad.vi"("Arcsec"=w297) -> ("rad"=w295:dbl)
                    n295 = global write "Global_Telescopio.vi" "Calagem AH"(w298) -> ()
                    n296 = global write "Global_Telescopio.vi" "Calagem DEC"(w295) -> ()
                  }
                }
                n297 = global write "Global_Telescopio.vi" "CorrecaoMin"("CorrecaoMin") -> ()
                n298 = global write "Global_Telescopio.vi" "tel_sts1 Array"("tel_sts1") -> ()
              }
              frame #1 {
                n299 = case shown="True" "Conf. Instrumentos" {
                  frame False {
                  }
                  frame True {
                    n300 = stacked-sequence {
                      frame #0 {
                        n301 = local read "Instrumento"() -> (w302:u16)
                        n302 = local read "Tabela Instrumentos"() -> (w311:string[][])
                        n303 = Build Array(w302) -> (w306:u16[])
                        n304 = Number To Decimal String(number=w306) -> (decimal integer string=w304:string[])  [unwired: 1 in]
                        n305 = String To Path(string="C:\\TCS\\SETUP\\INSTRUMENTOS.DAT") -> (path=w315:path)
                        n306 = Build Array(w304) -> (w305:string[][])
                        n307 = String To Path(string="C:\\TCS\\SETUP\\INSTRUM_ESCOLHIDO.DAT") -> (path=w307:path)
                        n308 = Delete(path (use dialog)=w315) -> (deleted path=w314:path)  [unwired: 4 in, 2 out]
                        n309 = Transpose 2D Array(2D array=w305) -> (transposed array=w303:string[][])
                        n310 = Delete(path (use dialog)=w307) -> (deleted path=w308:path)  [unwired: 4 in, 2 out]
                        n311 = Path To String(path=w314) -> (string=w313:string)
                        n312 = Path To String(path=w308) -> (string=w309:string)
                        n313 = call "salvaexel.vi"("appended array"=w311, "file name p/ exell"=w313) -> ()  [unwired: 1 in, 1 out]
                        n314 = call "salvaexel.vi"("appended array"=w303, "file name p/ exell"=w309) -> ()  [unwired: 1 in, 1 out]
                      }
                      frame #1 {
                        # "Valores Instrumentos Auto Guider"
                        # "Recarrega Globais necessárias"
                        n315 = local read "Tabela Instrumentos"() -> (w347:string[][])
                        n316 = Index Array(array=w347, index (col)=0 ("disabled index (col)")) -> (element=w344:string[])  [unwired: 1 in]
                        n317 = global write "Global_Telescopio.vi" "Lista Instrumentos"(w344) -> ()
                        n318 = local read "Instrumento"() -> (w343:u16)
                        n319 = property on="Instrumento" class="Ring (strict)"("Strings []"=w344) -> ()  [unwired: 2 in, 2 out]
                        n320 = global write "Global_Telescopio.vi" "Instrum"(w343) -> ()
                        n321 = Index Array(array=w347, index (row)=w343) -> (element=w345:string[])  [unwired: 1 in]
                        n322 = Index Array(array=w345, index #1=1 ("index")) -> (element #1=w339:string, element #2=w335:string, element #3=w332:string, element #4=w329:string, element #5=w325:string, element #6=w323:string, element #7=w318:string, element #8=w316:string)  [unwired: 7 in]
                        n323 = global write "Global_Telescopio.vi" "Foco Instrumento"(w316) -> ()
                        n324 = call "point_to_comma.vi"("Lat_A"=w323) -> ("Saída"=w324:string)
                        n325 = call "point_to_comma.vi"("Lat_A"=w318) -> ("Saída"=w317:string)
                        n326 = call "Comma_to_Point.vi"("Lat_A"=w339) -> ("Saída"=w340:string)
                        n327 = call "Comma_to_Point.vi"("Lat_A"=w335) -> ("Saída"=w336:string)
                        n328 = call "Comma_to_Point.vi"("Lat_A"=w325) -> ("Saída"=w326:string)
                        n329 = Fract/Exp String To Number(string=w324) -> (number=w322:dbl)  [unwired: 3 in, 1 out]
                        n330 = Fract/Exp String To Number(string=w317) -> (number=w320:dbl)  [unwired: 3 in, 1 out]
                        n331 = call <vilib>:"Trim Whitespace.vi"("string"=w332) -> ("trimmed string"=w334:string)  [unwired: 1 in]
                        n332 = call <vilib>:"Trim Whitespace.vi"("string"=w329) -> ("trimmed string"=w331:string)  [unwired: 1 in]
                        n333 = call "Arcsec to Rad.vi"("Arcsec"=w322) -> ("rad"=w321:dbl)
                        n334 = call "Arcsec to Rad.vi"("Arcsec"=w320) -> ("rad"=w319:dbl)
                        n335 = call "Formata_Numeros.vi"("Formato ex-> 7.2"="7.2", "Valor num"=w340) -> ("resulting string"=w341:string)
                        n336 = call "Formata_Numeros.vi"("Formato ex-> 7.2"="7.2", "Valor num"=w336) -> ("resulting string"=w337:string)
                        n337 = call "Formata_Numeros.vi"("Formato ex-> 7.2"="5.3", "Valor num"=w326) -> ("resulting string"=w327:string)
                        n338 = global write "Global_Telescopio.vi" "CalagemDEC_Inicial"(w318) -> ()
                        n339 = To Upper Case(1:w334) -> (0:w333:string)
                        n340 = To Upper Case(1:w331) -> (0:w330:string)
                        n341 = global write "Global_Telescopio.vi" "Calagem AH"(w321) -> ()
                        n342 = global write "Global_Telescopio.vi" "Calagem DEC"(w319) -> ()
                        n343 = global write "Global_Telescopio.vi" "CalagemAH_Inicial"(w323) -> ()
                        n344 = global write "Global_Telescopio.vi" "rotator_def"(w341) -> ()
                        n345 = global write "Global_Telescopio.vi" "guide_nor"(w337) -> ()
                        n346 = global write "Global_Telescopio.vi" "guide_esp"(w333) -> ()
                        n347 = global write "Global_Telescopio.vi" "esc_placa"(w327) -> ()
                        n348 = global write "Global_Telescopio.vi" "guide_cas"(w330) -> ()
                      }
                      frame #2 {
                        n349 = disable-structure shown="Disabled" {
                          frame Disabled {
                            # "25/10/2012 - Teste: deve ser retirado"
                            n350 = case shown="True" "Case Constant\n(See Context Help) 4" {
                              frame False {
                              }
                              frame True {
                                # "Salva as Globais Calagem"
                                n351 = global read "Global_Telescopio.vi" "Calagem AH"() -> (w353:dbl)
                                n352 = global read "Global_Telescopio.vi" "Calagem DEC"() -> (w352:dbl)
                                n353 = call "Rad to Arcsec.vi"("Radiano"=w353) -> ("Arcsec"=w350:dbl)
                                n354 = call "Rad to Arcsec.vi"("Radiano"=w352) -> ("Arcsec"=w351:dbl)
                                n355 = Build Array(w350, w351) -> (w360:dbl[])
                                n356 = Number To Fractional String(number=w360, precision (6)=i16 8) -> (F-format string=w361:string[])  [unwired: 2 in]
                                n357 = Build Array(w361) -> (w355:string[][])
                                n358 = String To Path(string="C:\\TCS\\SETUP\\GLOBAIS_CALAGEM.DAT") -> (path=w356:path)
                                n359 = Transpose 2D Array(2D array=w355) -> (transposed array=w354:string[][])
                                n360 = Delete(path (use dialog)=w356) -> (deleted path=w357:path)  [unwired: 4 in, 2 out]
                                n361 = Path To String(path=w357) -> (string=w358:string)
                                n362 = call "salvaexel.vi"("appended array"=w354, "file name p/ exell"=w358) -> ()  [unwired: 1 in, 1 out]
                              }
                            }
                          }
                          frame Enabled {
                          }
                        }
                      }
                    }
                  }
                }
              }
            }
          }
          frame "Utils" {
            n363 = stacked-sequence {
              frame #0 {
                (unwired) FALSE ("True = hora")
                n364 = global read "Global_Telescopio.vi" "Azimute GRAUS"() -> (→"Azimute":dbl)
                n365 = global read "Global_Telescopio.vi" "Zenital angle GRAUS"() -> (→"Ângulo Zenital":dbl)
                n366 = call <vilib>:"Trim Whitespace.vi"("string"="Dest Dec") -> ("trimmed string"=w370:string)  [unwired: 1 in]
                n367 = call <vilib>:"Trim Whitespace.vi"("string"="Hour Angle") -> ("trimmed string"=w367:string)  [unwired: 1 in]
                n368 = call "Comma_to_Point.vi"("Lat_A"=w370) -> ("Saída"=w369:string)
                n369 = call "Comma_to_Point.vi"("Lat_A"=w367) -> ("Saída"=w365:string)
                n370 = call "hms_rad.vi"("Texto Graus"=w369) -> ("radianos"=→"DestDEC":dbl)  [unwired: 4 in]
                n371 = call "hms_rad.vi"("True = hora"=TRUE, "Texto Graus"=w365) -> ("radianos"=→"DestAH":dbl)  [unwired: 3 in]
              }
              frame #1 {
                n372 = case shown="True" "SALVA CONFIG" {
                  frame False {
                  }
                  frame True {
                    n373 = local read "Raio Máximo"() -> (w402:dbl)
                    n374 = local read "Limite Oeste"() -> (w389:dbl)
                    n375 = local read "Limite Leste"() -> (w390:dbl)
                    n376 = local read "DestAH"() -> (w408:dbl)
                    n377 = local read "DestCUP"() -> (w409:i32)
                    n378 = local read "Z_Segurança"() -> (w405:dbl)
                    n379 = local read "Z_Libera"() -> (w404:dbl)
                    n380 = local read "DestDEC"() -> (w407:dbl)
                    n381 = local read "Z_Max"() -> (w403:dbl)
                    n382 = global write "Global_Telescopio.vi" "Raio Máximo"(w402) -> ()
                    n383 = global write "Global_Telescopio.vi" "Limite EAST"(w390) -> ()
                    n384 = global write "Global_Telescopio.vi" "Limite WEST"(w389) -> ()
                    n385 = global write "Global_Telescopio.vi" "DestAH"(w408) -> ()
                    n386 = global write "Global_Telescopio.vi" "DestDEC"(w407) -> ()
                    n387 = global write "Global_Telescopio.vi" "DestCUP"(w409) -> ()
                    n388 = local read "Tempo delay"() -> (w388:i32)
                    n389 = global write "Global_Telescopio.vi" "Tempo delay"(w388) -> ()
                    n390 = local read "Hora vent inicial"() -> (w379:i32)
                    n391 = local read "Tempo Atualização All Sky"() -> (w391:i32)
                    n392 = local read "Tempo Atualização Cam 0"() -> (w392:i32)
                    n393 = local read "Tempo Atualização Cam 1"() -> (w393:i32)
                    n394 = local read "Tempo Atualização Cam 2"() -> (w394:i32)
                    n395 = local read "Tempo Atualização Cam 3"() -> (w395:i32)
                    n396 = global write "Global_Telescopio.vi" "Tempo Atulização Cam 0"(w392) -> ()
                    n397 = global write "Global_Telescopio.vi" "Tempo Atulização Cam 1"(w393) -> ()
                    n398 = global write "Global_Telescopio.vi" "Tempo Atulização Cam 2"(w394) -> ()
                    n399 = global write "Global_Telescopio.vi" "Tempo Atulização Cam 3"(w395) -> ()
                    n400 = global write "Global_Telescopio.vi" "Tempo Atulização All Sky"(w391) -> ()
                    n401 = local read "Hora vent final"() -> (w378:i32)
                    n402 = Number To Decimal String(number=w379) -> (decimal integer string=w377:string)  [unwired: 1 in]
                    n403 = Number To Decimal String(number=w378) -> (decimal integer string=w376:string)  [unwired: 1 in]
                    n404 = local read "habilita supervisao"() -> (w387:bool)
                    n405 = global write "Global_Telescopio.vi" "Habilita supervisao"(w387) -> ()
                    n406 = global write "Global_Telescopio.vi" "Hora vent inicial"(w377) -> ()
                    n407 = local read "Enable ventilador"() -> (w384:bool)
                    n408 = global write "Global_Telescopio.vi" "Enable ventilador"(w384) -> ()
                    n409 = global write "Global_Telescopio.vi" "Hora vent final"(w376) -> ()
                    n410 = local read "Caminho camera"() -> (w380:string)
                    n411 = global write "Global_Telescopio.vi" "Caminho camera"(w380) -> ()
                    n412 = case shown="True" w387 {
                      tunnel: [0 1] -> w386
                      frame False {
                      }
                      frame True {
                      }
                    }
                    n413 = case shown="True" w384 {
                      tunnel: [0 1] -> w385
                      frame False {
                      }
                      frame True {
                      }
                    }
                    n414 = Build Array(w408, w407, w409, w405, w404, w403, w402, w390, w389, w391, w392, w393, w394, w395, w388, w386, w385) -> (w414:dbl[])
                    n415 = Number To Fractional String(number=w414, precision (6)=i16 8) -> (F-format string=w382:string[])  [unwired: 2 in]
                    n416 = String To Path(string="C:\\TCS\\SETUP\\Utils.txt") -> (path=w412:path)
                    n417 = local read "Tabela Proteção"() -> (w396:string[][])
                    n418 = String To Path(string="C:\\TCS\\SETUP\\TABELA_PROTE敲O.DAT") -> (path=w399:path)
                    n419 = Delete(path (use dialog)=w399) -> (deleted path=w400:path)  [unwired: 4 in, 2 out]
                    n420 = global write "Global_Telescopio.vi" "Tabela Proteção"(w396) -> ()
                    n421 = Delete(path (use dialog)=w412) -> (deleted path=w411:path)  [unwired: 4 in, 2 out]
                    n422 = Path To String(path=w400) -> (string=w401:string)
                    n423 = Transpose 2D Array(2D array=w396) -> (transposed array=w398:string[][])
                    n424 = Path To String(path=w411) -> (string=w410:string)
                    n425 = local read "Senha LEAF"() -> (w375:string)
                    n426 = Build Array (concatenate)(w382, w380, w377, w376, w375) -> (w381:string[])
                    n427 = Build Array(w381) -> (w383:string[][])
                    n428 = Transpose 2D Array(2D array=w383) -> (transposed array=w413:string[][])
                    n429 = global write "Global_Telescopio.vi" "Senha LEAF"(w375) -> ()
                    n430 = call "salvaexel.vi"("appended array"=w398, "file name p/ exell"=w401) -> ()  [unwired: 1 in, 1 out]
                    n431 = call "salvaexel.vi"("appended array"=w413, "file name p/ exell"=w410) -> ()  [unwired: 1 in, 1 out]
                  }
                }
              }
              frame #2 {
                n432 = case shown="True" "Download_Finals2000A.all" {
                  selector: "Download_Finals2000A.all" -> [w422 w425]
                  tunnel: [w422 FALSE] -> w420
                  frame False {
                  }
                  frame True {
                    n433 = flat-sequence {
                      tunnel: w425 -> [w427]
                      tunnel: [w427] -> w423
                      tunnel: w423 -> [w430]
                      frame #0 {
                        n434 = local write "DownloadOK"(FALSE) -> ()
                      }
                      frame #1 {
                        (unwired) "http://maia.usno.navy.mil/ser7/finals2000A.all" ("URL")
                        (unwired) "http://toshi.nofs.navy.mil/ser7/finals2000A.all" ("URL")
                        # "http://maia.usno.navy.mil/ser7/finals2000A.all\nna pasta C:\\TCS\\ARQUIVOS\\"
                        n435 = local write "DownloadWait"(w430) -> ()
                        n436 = property on="DownloadWait" class="Bool (strict)"("Blinking"=w430) -> ()  [unwired: 2 in, 2 out]
                        n437 = property on="DownloadWait" class="Bool (strict)"("Visible"=w430) -> ()  [unwired: 2 in, 2 out]
                        n438 = String To Path(string="C:\\TCS\\ARQUIVOS\\finals2000A.all" ("URL")) -> (path=w432:path)
                        n439 = call "URL Get Document.vi"("file path (NAP)"=w432, "URL"="URL do finals2000A.all:") -> ("success"=→"DownloadOK":bool)  [unwired: 5 in, 4 out]
                      }
                    }
                  }
                }
                "DownloadWait" <- w420
                n440 = property on="DownloadWait" class="Bool (strict)"("Blinking"=w420) -> ()  [unwired: 2 in, 2 out]
                n441 = property on="DownloadWait" class="Bool (strict)"("Visible"=w420) -> ()  [unwired: 2 in, 2 out]
              }
            }
          }
        }
        n442 = Wait Until Next ms Multiple(millisecond multiple=u32 200) -> ()  [unwired: 1 out]
      }
    }
    frame #2 {
    }
  }
